vi "Close.vi"(8 "error in (no error)":errorcluster, 11 "ModbusSp in":refnum<class "ModbusSp.lvclass">) -> (0 "error out":errorcluster, 3 "ModbusSp out":refnum<class "ModbusSp.lvclass">)   [LabVIEW 2019, in "ModbusSp.lvclass"]
uses:
  ModbusSp.lvclass
  ModbusSp.lvclass/ModbusSp.ctl
  <vilib>/NI/Modbus Library/API/Slave/Modbus Slave.lvclass
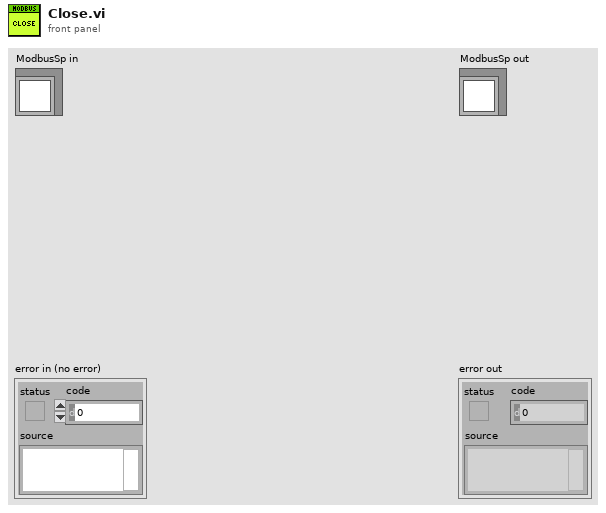
[diagram p1: front panel]
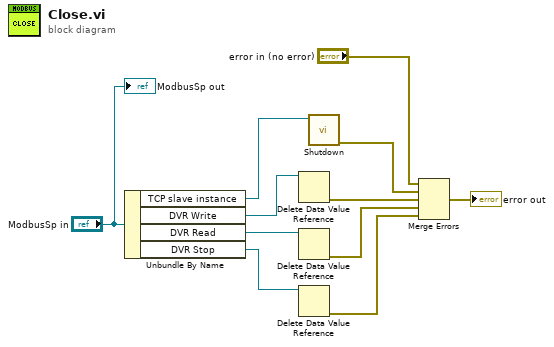
[diagram p0: block diagram]
diagram:
  n1 = Unbundle By Name("ModbusSp in") -> ("TCP slave instance"=w7:refnum<class "Modbus Slave.lvclass">, "DVR Write"=w10:refnum<data-value>, "DVR Read"=w9:refnum<data-value>, "DVR Stop"=w8:refnum<data-value>)
  n2 = Delete Data Value Reference(data value reference=w10) -> (error out=w4:errorcluster)  [unwired: 1 in, 1 out]
  n3 = Delete Data Value Reference(data value reference=w9) -> (error out=w5:errorcluster)  [unwired: 1 in, 1 out]
  n4 = Delete Data Value Reference(data value reference=w8) -> (error out=w6:errorcluster)  [unwired: 1 in, 1 out]
  n5 = call-dynamic "Shutdown.vi"("Modbus slave in"=w7) -> ("error out"=w3:errorcluster)  [unwired: 10 in]
  n6 = Merge Errors("error in (no error)", w3, w4, w5, w6) -> (→"error out":errorcluster)
  "ModbusSp out" <- "ModbusSp in"
